vi "Event-Toolbar.vi"(5 "Menu ref.":refnum<k9>, 7 "Tag":string, 8 "error in (no error)":errorcluster, 10 "Data ref. in":refnum<data-value>, 11 "UI ref. in":refnum<data-value>) -> (0 "error out":errorcluster, 2 "Data ref.":refnum<data-value>, 3 "UI ref.":refnum<data-value>)   [LabVIEW 2013, in "CameraVision.lvlib" / "CV-UI.lvclass"]
uses:
  CV-UI.lvclass
  Main/CV-Main.lvclass
  Panes/Pane-names.ctl
  CV-UI.lvclass/CV-UI.ctl
  Read Panes.vi
  Panes/CV-Panes.lvclass
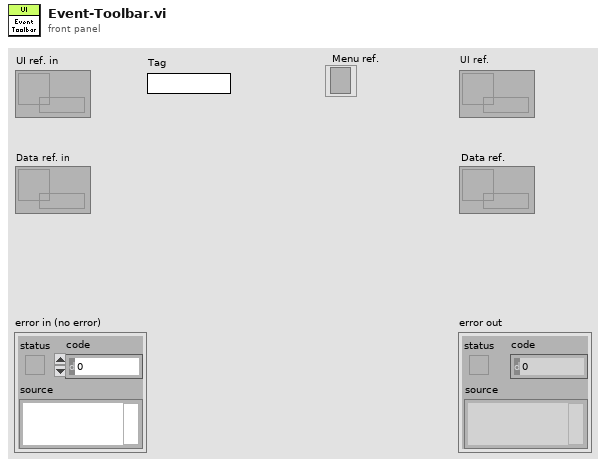
[diagram p1: front panel]
types:
  T1 = typedef "CameraVision.lvlib/CV-Panes.lvclass/Pane-names.ctl" = enum16{"Toolbar", "Help bar", "Toolbar lower border", "Settings", "Displays", "Status bar upper border", "General state bar", "Information bar"}
  T2 = typedef "CameraVision.lvlib/CV-Panes.lvclass/Object-reference.ctl" = refnum<data-value>
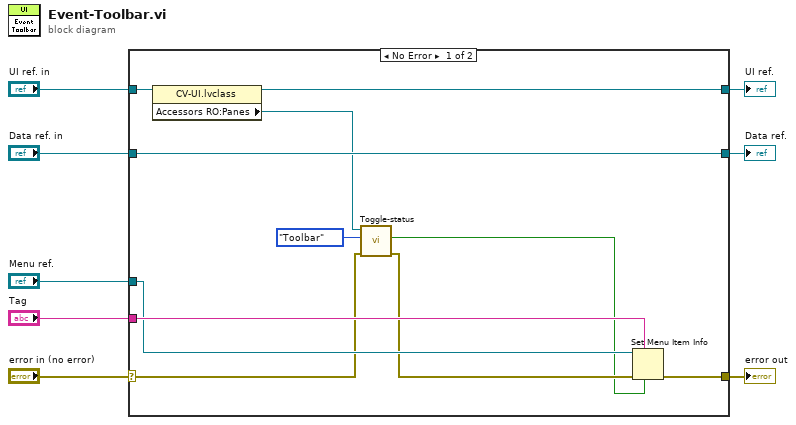
[diagram p0: block diagram]
diagram:
  n1 = case shown="No Error" "error in (no error)" {
    selector: "error in (no error)" -> [w12 w22]
    tunnel: [w9 w22] -> w7
    tunnel: [w14 w21] -> w5
    tunnel: "UI ref. in" -> [w15 w21]
    tunnel: "Data ref. in" -> [w19 w20]
    tunnel: "Tag" -> [w18 _]
    tunnel: [w19 w20] -> w3
    tunnel: "Menu ref." -> [w17 _]
    frame No Error {
      n2 = property class="CV-UI.lvclass"(reference=w15) -> (reference out=w14:refnum<data-value>, "Accessors RO:Panes"=w13:T2)  [unwired: 1 in, 1 out]
      n3 = call "Toggle-status.vi"("error in (no error)"=w12, "Pane"=Pane-names."Toolbar", "Panes in"=w13) -> ("error out"=w11:errorcluster, "Status"=w10:bool)  [unwired: 6 in, 1 out]
      n4 = Set Menu Item Info(6:w10, 7:w18, 8:w11, 11:w17) -> (0:w9:errorcluster)  [unwired: 3 in, 1 out]
    }
    frame Error {
    }
  }
  "error out" <- w7
  "Data ref." <- w3
  "UI ref." <- w5
